vi "FESTO CTEU-EP TO VTUG Basic MODBUS over TCPIP.vi"() -> ()   [LabVIEW 2018]
doc: "Use this template to build a simple state machine design pattern. Each state executes code and determines which state to transition to."
uses:
  controls/State.ctl
  controls/Data.ctl
  <vilib>/NI/Modbus Library/API/Wrapper/Create TCP Master.vi
  <vilib>/NI/Modbus Library/API/Master/Modbus Master.lvclass
  <vilib>/NI/Modbus Library/API/Wrapper/API Main.lvlib
panel:
  out "Sent Value":i32
  in  "Cylinder 4":bool
  in  "Cylinder 3":bool
  in  "Cylinder 2":bool
  in  "Cylinder 1":bool
  in  "stop":bool
  out "Current register values":u16[](array[numeric])
  in  "PORT":i16=502
  in  "Slave Address":string="192.168.1.7"
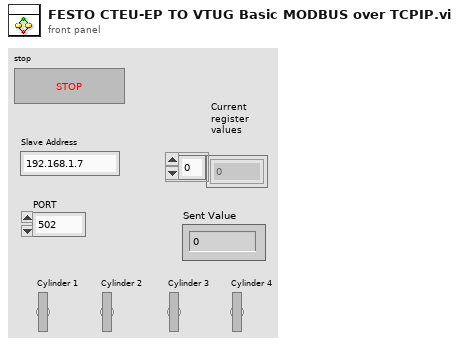
[diagram p1: front panel]
types:
  T1 = typedef "Data.ctl" = cluster{"Boolean <Replace Me>":bool, "String <Replace Me>":string, "Numeric <Replace Me>":dbl}
  T2 = typedef "State.ctl" = enum16{"Initialize", "Wait for Event", "Write to Register", "Read From Register", "Exit"}
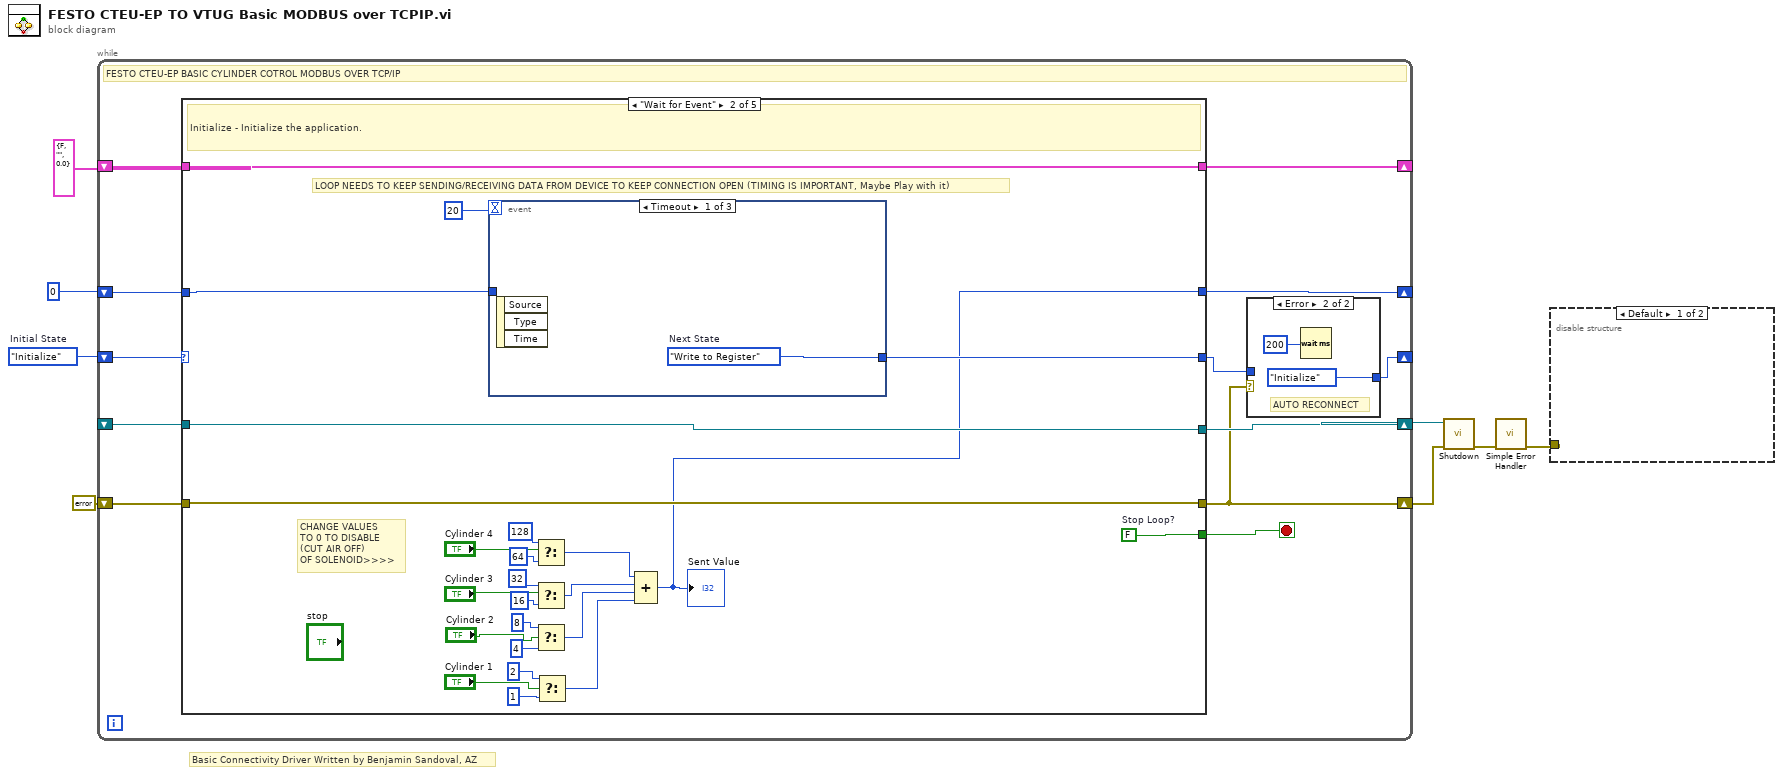
[diagram p0: block diagram]
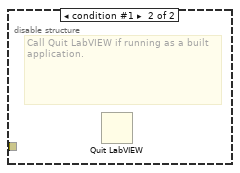
[diagram p2: hidden frame]
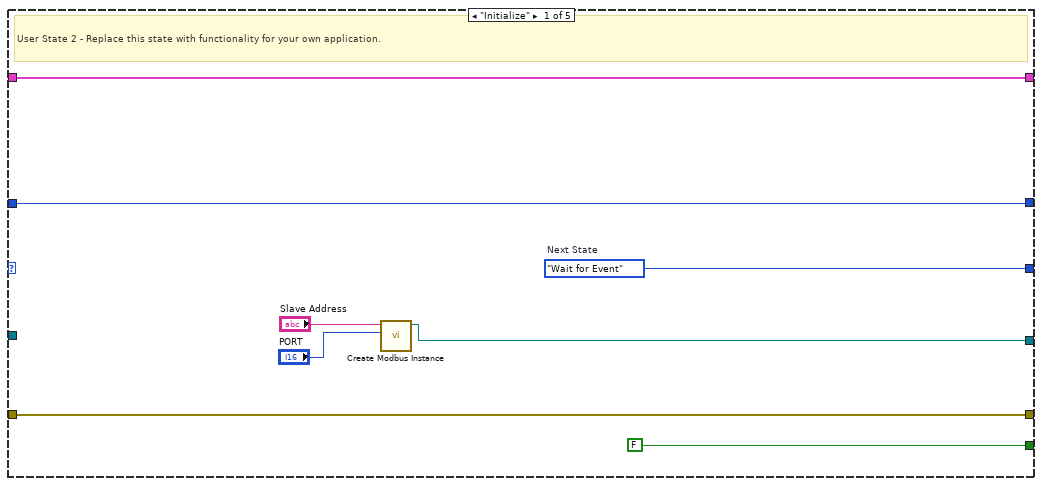
[diagram p4: hidden frame]
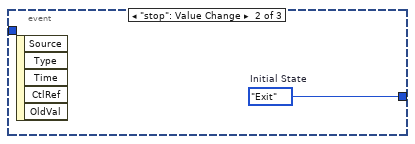
[diagram p5: hidden frame]
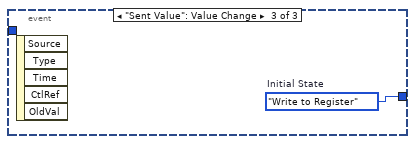
[diagram p6: hidden frame]
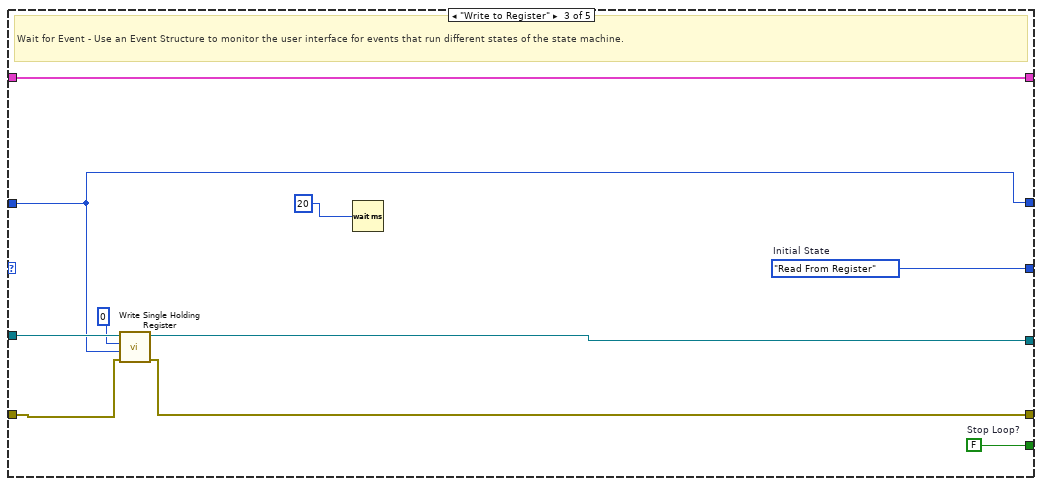
[diagram p7: hidden frame]
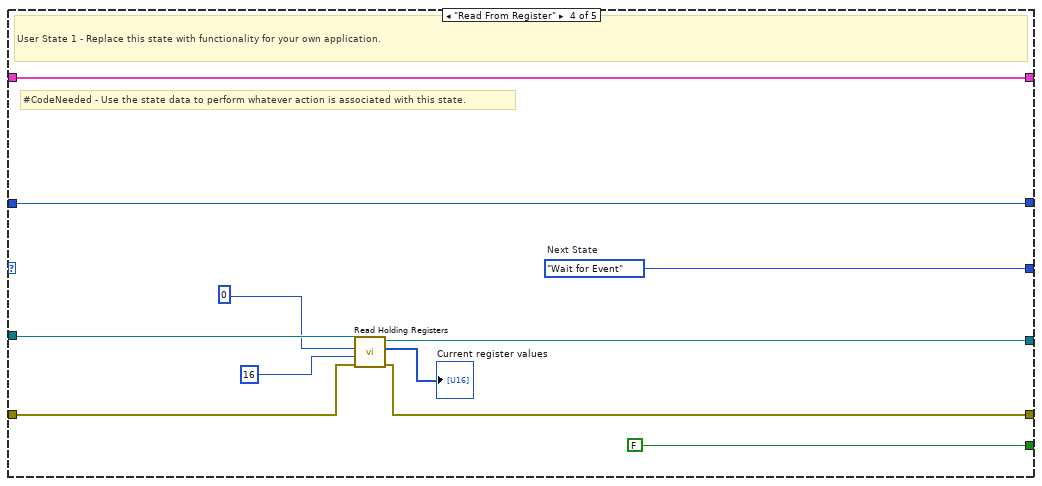
[diagram p8: hidden frame]
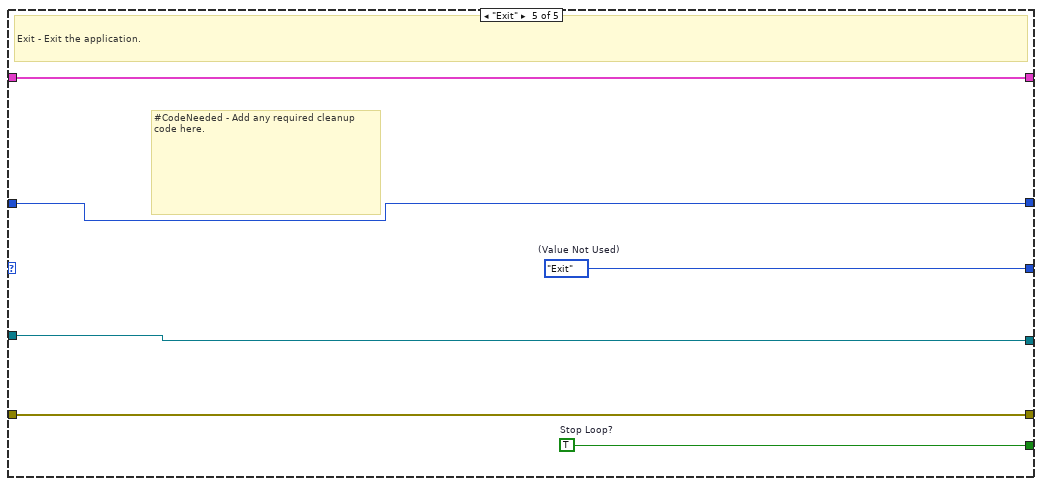
[diagram p9: hidden frame]
diagram:
  w8 = State."Initialize"  # Initial State
  # "Basic Connectivity Driver Written by Benjamin Sandoval, AZ"
  n1 = while {
    shift-right: [w12] -> _
    shift-left: w8 -> [w20]
    shift-right: [w18] -> _
    shift-left: T1 {"Boolean <Replace Me>"=FALSE, "String <Replace Me>"="", "Numeric <Replace Me>"=0.0} ("Data") -> [w19]
    shift-right: [w9] -> w2
    shift-left: errorcluster {"status"=FALSE, "code"=0, "source"=""} ("error constant") -> [w17]
    shift-right: [w15] -> w3
    shift-left: _ -> [w16]
    shift-right: [w14] -> _
    shift-left: 0 -> [w13]
    stop <- w10 stop-if-true
    # "FESTO CTEU-EP BASIC CYLINDER COTROL MODBUS OVER TCP/IP"
    n2 = case shown="\"Wait for Event\"" w20 {
      tunnel: [w31 w50 w66 w79 w85] -> w11
      tunnel: [FALSE ("Stop Loop?") w55 w68 FALSE ("Stop Loop?") w83] -> w10
      tunnel: w19 -> [w29 w53 w67 w77 w84]
      tunnel: [w29 w53 w67 w77 w84] -> w18
      tunnel: w17 -> [w28 w54 w63 w74 w82]
      tunnel: [w28 w54 w62 w73 w82] -> w9
      tunnel: w16 -> [_ w52 w65 w76 w81]
      tunnel: [w24 w52 w64 w75 w81] -> w15
      tunnel: [w27 w32 w59 w69 w80] -> w14
      tunnel: w13 -> [w27 w49 w59 w69 w80]
      frame "Initialize" {
        w31 = State."Wait for Event"  # Next State
        # "User State 2 - Replace this state with functionality for your own application."
        n3 = call-poly <vilib>:"Create Modbus Instance.vi"("port (502)"="PORT", "address"="Slave Address") -> ("TCP master instance"=w24:refnum<class "Modbus Master.lvclass">)  [unwired: 8 in, 1 out]
      }
      frame "Wait for Event" {
        w55 = FALSE  # Stop Loop?
        # "LOOP NEEDS TO KEEP SENDING/RECEIVING DATA FROM DEVICE TO KEEP CONNECTION OPEN (TIMING IS IMPORTANT, Maybe Play with it)"
        # "CHANGE VALUES\nTO 0 TO DISABLE\n(CUT AIR OFF)\nOF SOLENOID>>>>"
        # "Initialize - Initialize the application."
        n4 = event shown="[0] Timeout" {
          selector: _ -> [_ _ _]
          dyn-events: _ -> [_ _ _]
          timeout: 20 -> [_ _ _]
          tunnel: [w56 w57 w58] -> w50
          tunnel: w49 -> [_ _ _]
          event Timeout {
            w56 = State."Write to Register"  # Next State
            n5 = event-data() -> ()  [unwired: 1 in, 3 out]
          }
          event "stop": Value Change {
            w57 = State."Exit"  # Initial State
            n6 = event-data() -> ()  [unwired: 1 in, 5 out]
          }
          event "Sent Value": Value Change {
            w58 = State."Write to Register"  # Initial State
            n7 = event-data() -> ()  [unwired: 1 in, 5 out]
          }
        }
        n8 = Select(t=128, s="Cylinder 4", f=64) -> (s? t:f=w36:i32)
        n9 = Select(t=32, s="Cylinder 3", f=16) -> (s? t:f=w35:i32)
        n10 = Select(t=8, s="Cylinder 2", f=4) -> (s? t:f=w34:i32)
        n11 = Select(t=2, s="Cylinder 1", f=1) -> (s? t:f=w33:i32)
        n12 = Compound Arithmetic op=ADD(w36, w35, w34, w33) -> (w32:i32)
        "Sent Value" <- w32
      }
      frame "Write to Register" {
        w66 = State."Read From Register"  # Initial State
        w68 = FALSE  # Stop Loop?
        # "Wait for Event - Use an Event Structure to monitor the user interface for events that run different states of the state machine."
        n13 = call-dynamic "Write Single Holding Register.vi"("error in"=w63, "register to write"=w59, "address"=0, "Modbus master in"=w65) -> ("error out"=w62:errorcluster, "Modbus master out"=w64:refnum<class "Modbus Master.lvclass">)  [unwired: 6 in]
        n14 = Wait (ms)(milliseconds to wait=20) -> ()  [unwired: 1 out]
      }
      frame "Read From Register" {
        w79 = State."Wait for Event"  # Next State
        # "#CodeNeeded - Use the state data to perform whatever action is associated with this state."
        # "User State 1 - Replace this state with functionality for your own application."
        n15 = call-dynamic "Read Holding Registers.vi"("error in"=w74, "number of inputs"=16, "starting address"=0, "Modbus master in"=w76) -> ("error out"=w73:errorcluster, "register values"=→"Current register values":u16[], "Modbus master out"=w75:refnum<class "Modbus Master.lvclass">)  [unwired: 5 in]
      }
      frame "Exit" {
        w83 = TRUE  # Stop Loop?
        w85 = State."Exit"  # (Value Not Used)
        # "#CodeNeeded - Add any required cleanup code here."
        # "Exit - Exit the application."
      }
    }
    n16 = case shown="Error" w9 {
      tunnel: w11 -> [w21 _]
      tunnel: [w21 State."Initialize" ("Initial State")] -> w12
      frame No Error {
      }
      frame Error {
        # "AUTO RECONNECT"
        n17 = Wait (ms)(milliseconds to wait=200) -> ()  [unwired: 1 out]
      }
    }
  }
  n18 = call-dynamic "Shutdown.vi"("error in"=w2, "Modbus master in"=w3) -> ("error out"=w1:errorcluster)  [unwired: 9 in]
  n19 = call <vilib>:"Simple Error Handler.vi"("error in (no error)"=w1) -> ("error out"=w5:errorcluster)  [unwired: 4 in, 4 out]
  n20 = disable-structure shown="Default" {
    disable-tunnel: w5 -> [_ _]
    frame condition #0 (active) {
    }
    frame condition #1 {
      # "Call Quit LabVIEW if running as a built application."
      n21 = Quit LabVIEW() -> ()  [unwired: 1 in]
    }
  }
